vi "Check.vi"(0 "BroadcastRegistry in":refnum<class "BroadcastRegistry.lvclass">, 5 "Status":string, 7 "Source":string, 11 "Target":string) -> (4 "BroadcastRegistry out":refnum<class "BroadcastRegistry.lvclass">, 6 "Response Message Info":string[](array[string]))   [LabVIEW 2020, in "Communicable State Machine.lvlib" / "BroadcastRegistry.lvclass"]
uses:
  BroadcastRegistry.lvclass
  BroadcastRegistry.lvclass/BroadcastRegistry.ctl
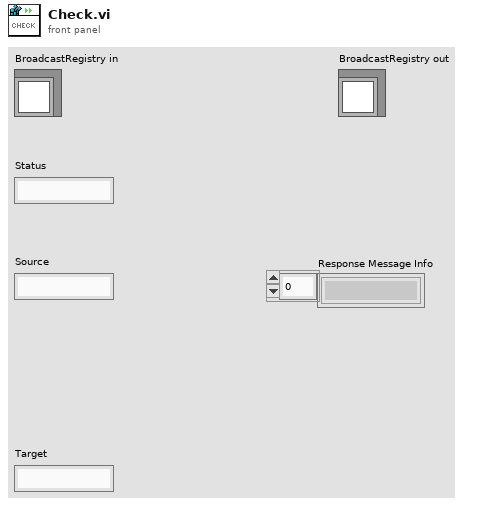
[diagram p1: front panel]
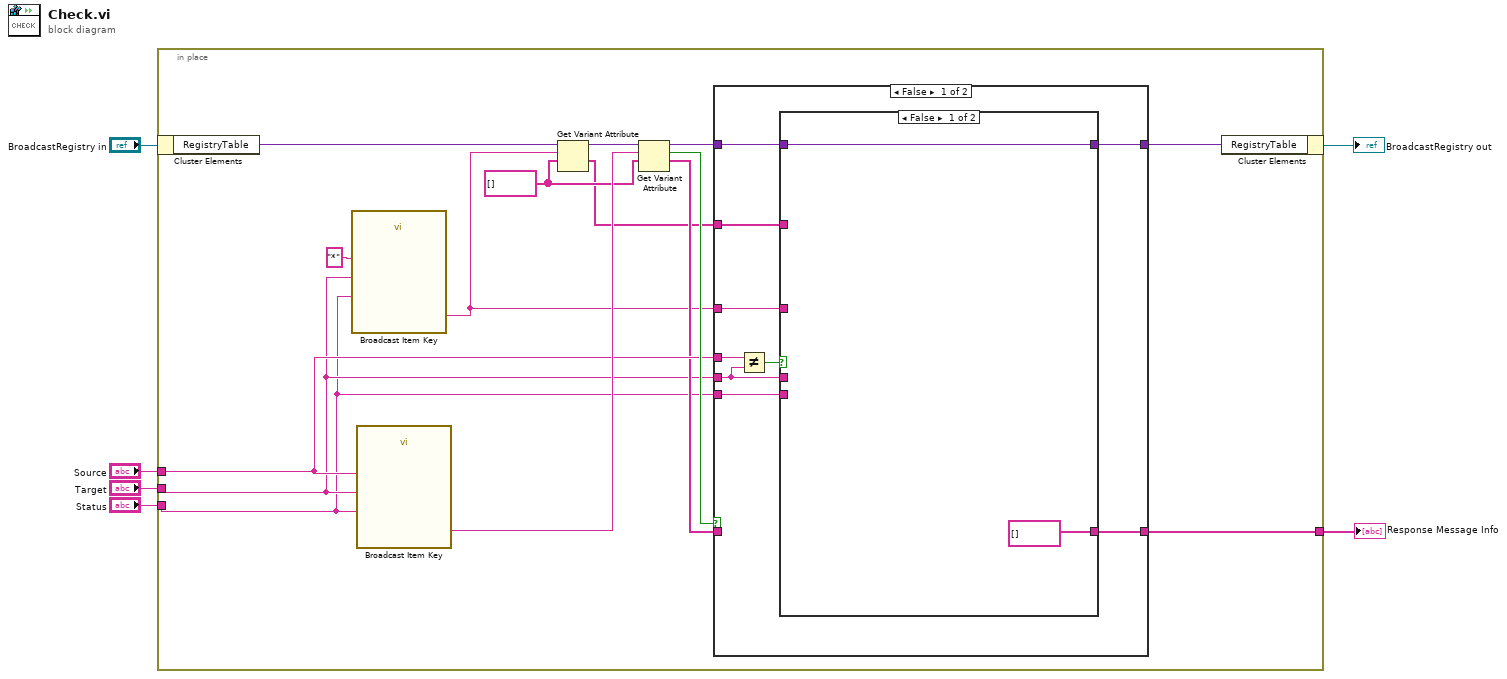
[diagram p0: block diagram]
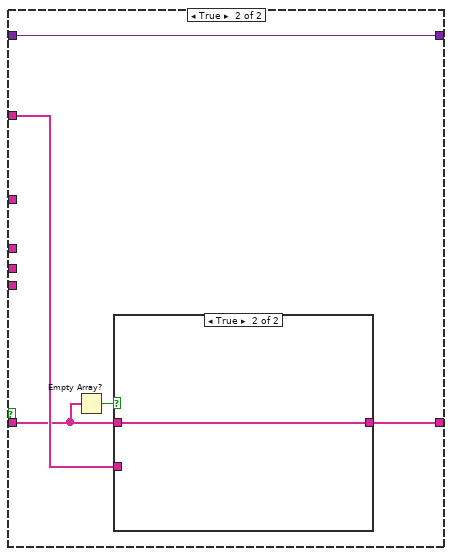
[diagram p3: hidden frame]
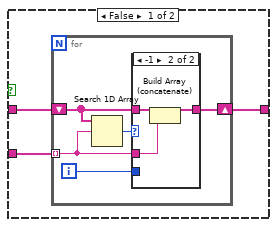
[diagram p4: hidden frame]
diagram:
  n1 = in-place {
    in-place-border: "Status" -> [w12]
    in-place-border: "Target" -> [w13]
    in-place-border: "Source" -> [w17]
    in-place-border: [w16] -> w1
    w8 = string[] [] ("Response Message Info")
    n2 = in-place-cluster #1("BroadcastRegistry in") -> ("RegistryTable"=w11:variant)
    n3 = call "Broadcast Item Key.vi"("status"=w12, "target"=w13, "source"="*" ("Source")) -> ("key"=w9:string)  [unwired: 2 in]
    n4 = call "Broadcast Item Key.vi"("status"=w12, "target"=w13, "source"=w17) -> ("key"=w21:string)  [unwired: 2 in]
    n5 = Get Variant Attribute(Variant=w11, name=w9, default value (empty Variant)=w8) -> (duplicate Variant=w10:variant, value=w7:string[])  [unwired: 1 in, 2 out]
    n6 = Get Variant Attribute(Variant=w10, name=w21, default value (empty Variant)=w8) -> (duplicate Variant=w20:variant, found=w19:bool, value=w15:string[])  [unwired: 1 in, 1 out]
    n7 = case shown="False" w19 {
      tunnel: w12 -> [w30 _]
      tunnel: w13 -> [w25 _]
      tunnel: w20 -> [w29 w39]
      tunnel: [w28 w39] -> w18
      tunnel: w15 -> [_ w36]
      tunnel: [w27 w37] -> w16
      tunnel: w17 -> [w26 _]
      tunnel: w9 -> [w23 _]
      tunnel: w7 -> [w22 w38]
      frame False {
        n8 = Not Equal?(x=w26, y=w25) -> (x != y?=w24:bool)
        n9 = case shown="False" w24 {
          tunnel: w30 -> [_ _]
          tunnel: w25 -> [_ _]
          tunnel: w29 -> [w32 w34]
          tunnel: [w32 w34] -> w28
          tunnel: [string[] [] ("Response Message Info") w33] -> w27
          tunnel: w23 -> [_ _]
          tunnel: w22 -> [_ w33]
          frame False {
          }
          frame True {
          }
        }
      }
      frame True {
        n10 = Empty Array?(array=w36) -> (empty?=w35:bool)
        n11 = case shown="True" w35 {
          tunnel: w38 -> [w42 _]
          tunnel: [w41 w52] -> w37
          tunnel: w36 -> [w40 w52]
          frame False {
            n12 = for {
              tunnel: w42 -> [w46] mode=indexing
              shift-right: [w45] -> w41
              shift-left: w40 -> [w44]
              i -> [w43]
              n13 = Search 1D Array(1D array=w44, element=w46) -> (index of element=w47:i32)  [unwired: 1 in]
              n14 = case shown="-1" w47 {
                tunnel: w46 -> [_ w51]
                tunnel: [w48 w49] -> w45
                tunnel: w44 -> [w48 w50]
                tunnel: w43 -> [_ _]
                frame Default {
                }
                frame -1 {
                  n15 = Build Array (concatenate)(w50, w51) -> (w49:string[])
                }
              }
            }
          }
          frame True {
          }
        }
      }
    }
    n16 = in-place-cluster #1("RegistryTable"=w18) -> (→"BroadcastRegistry out":refnum<class "BroadcastRegistry.lvclass">)
  }
  "Response Message Info" <- w1
